vi "DeleteAllErrors.vi"(11 "path":path) -> ()   [LabVIEW 2012]
panel:
  out "error out":errorcluster
  in  "error in (no error)":errorcluster
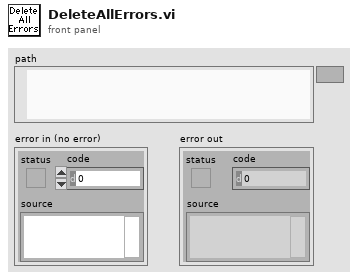
[diagram p1: front panel]
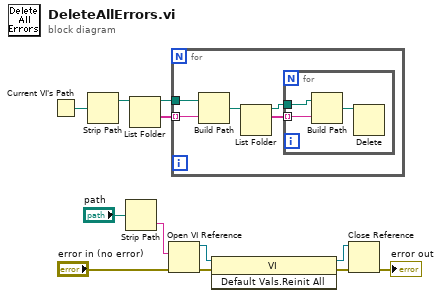
[diagram p0: block diagram]
diagram:
  n1 = Current VI's Path() -> (path=w12:path)
  n2 = Strip Path(path=w12) -> (stripped path=w11:path)  [unwired: 1 out]
  n3 = Strip Path(path="path") -> (name=w7:string)  [unwired: 1 out]
  n4 = List Folder(path=w11) -> (path out=w10:path, folder names=w9:string[])  [unwired: 3 in, 2 out]
  n5 = Open VI Reference(vi path=w7, error in (no error)="error in (no error)") -> (vi reference=w8:refnum<vi>, error out=w4:errorcluster)  [unwired: 4 in]
  n6 = for {
    tunnel: w10 -> [w16]
    tunnel: w9 -> [w15] mode=indexing
    n7 = Build Path(base path=w16, name or relative path=w15) -> (appended path=w17:path)
    n8 = List Folder(path=w17) -> (path out=w14:path, filenames=w13:string[])  [unwired: 3 in, 2 out]
    n9 = for {
      tunnel: w14 -> [w20]
      tunnel: w13 -> [w19] mode=indexing
      n10 = Build Path(base path=w20, name or relative path=w19) -> (appended path=w18:path)
      n11 = Delete(path (use dialog)=w18) -> ()  [unwired: 4 in, 3 out]
    }
  }
  n12 = invoke class="VI" method="Default Vals.Reinit All"(reference=w8, error in=w4) -> (reference out=w6:refnum<vi>, error out=w3:errorcluster)  [unwired: 1 in, 1 out]
  n13 = Close Reference(reference=w6, error in (no error)=w3) -> (error out=→"error out":errorcluster)
